vi "Load-Lookup Icon.vi"(8 "error in (no error)":errorcluster, 10 "Shell Icon":T1, 11 "TreeDirectory in":refnum<class "TreeDirectory.lvclass">) -> (0 "error out":errorcluster, 2 "Icon Index":i32, 3 "TreeDirectory (dup)":refnum<class "TreeDirectory.lvclass">)   [LabVIEW 2015, in "TreeDirectory.lvclass"]
uses:
  TreeDirectory.lvclass
  <vilib>/picture/picture.llb/imagedata.ctl
  TreeDirectory.lvclass/TreeDirectory.ctl
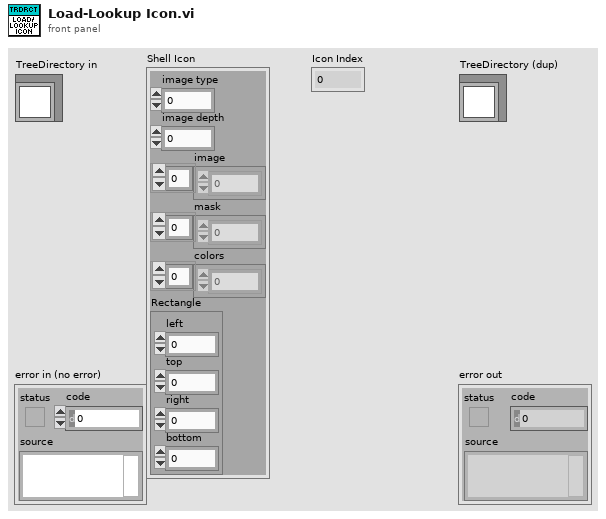
[diagram p1: front panel]
types:
  T1 = typedef "imagedata.ctl" = cluster{"image type":i32, "image depth":i32, "image":u8[], "mask":u8[], "colors":u32[], "Rectangle":cluster{"left":i16, "top":i16, "right":i16, "bottom":i16}}
  T2 = typedef "TreeDirectory.lvclass/State Data.ctl" = cluster{"IconLibrary":variant}
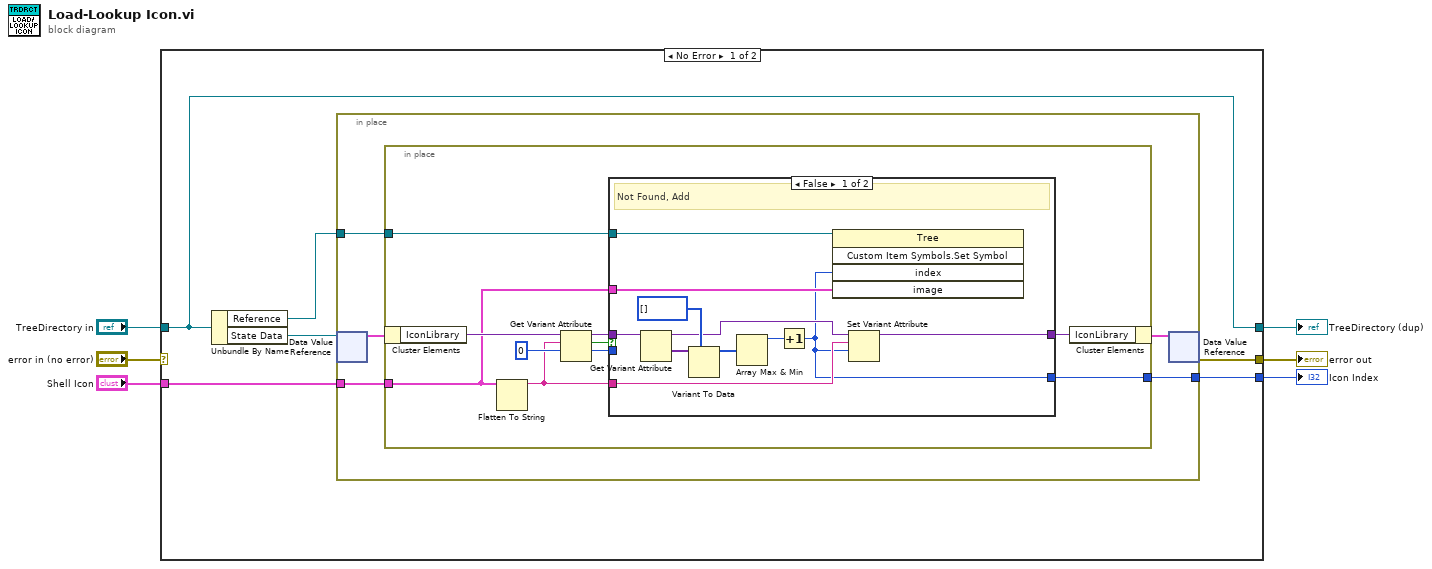
[diagram p0: block diagram]
diagram:
  n1 = case shown="No Error" "error in (no error)" {
    selector: "error in (no error)" -> [_ w42]
    tunnel: [w10 w42] -> w5
    tunnel: [w7 w41] -> w3
    tunnel: "TreeDirectory in" -> [w7 w41]
    tunnel: "Shell Icon" -> [w12 _]
    tunnel: [w11 _] -> w1
    frame No Error {
      n2 = Unbundle By Name(w7) -> ("Reference"=w8:refnum<vi>, "State Data"=w9:refnum<data-value>)
      n3 = in-place {
        in-place-border: w12 -> [w16]
        in-place-border: [w15] -> w11
        in-place-border: w8 -> [w13]
        n4 = in-place-dvr #1(w9) -> (w17:T2)  [unwired: 1 out]
        n5 = in-place {
          in-place-border: w16 -> [w19]
          in-place-border: [w21] -> w15
          in-place-border: w13 -> [w20]
          n6 = in-place-cluster #2(w17) -> ("IconLibrary"=w27:variant)
          n7 = Flatten To String(anything=w19) -> (data string=w18:string)  [unwired: 3 in, 2 out]
          n8 = Get Variant Attribute(Variant=w27, name=w18, default value (empty Variant)=0) -> (duplicate Variant=w24:variant, found=w25:bool, value=w22:i32)  [unwired: 1 in, 1 out]
          n9 = case shown="False" w25 {
            tunnel: w24 -> [w38 w40]
            tunnel: [w30 w40] -> w23
            tunnel: w22 -> [_ w39]
            tunnel: [w28 w39] -> w21
            tunnel: w20 -> [w33 _]
            tunnel: w19 -> [w32 _]
            tunnel: w18 -> [w29 _]
            frame False {
              # "Not Found, Add"
              n10 = Get Variant Attribute(Variant=w38) -> (duplicate Variant=w34:variant, values=w37:variant[])  [unwired: 3 in, 2 out]
              n11 = Variant To Data(type=i32[] [], Variant=w37) -> (data=w35:i32[])  [unwired: 1 in, 1 out]
              n12 = Array Max & Min(array=w35) -> (max value=w31:i32)  [unwired: 3 out]
              n13 = Increment(x=w31) -> (x+1=w28:i32)
              n14 = invoke class="Tree" method="Custom Item Symbols.Set Symbol"(reference=w33, "index"=w28, "image"=w32) -> ()  [unwired: 2 in, 5 out]
              n15 = Set Variant Attribute(Variant=w34, name=w29, value=w28) -> (Variant out=w30:variant)  [unwired: 1 in, 2 out]
            }
            frame True {
              # "Found, Pass Index"
            }
          }
          n16 = in-place-cluster #2("IconLibrary"=w23) -> (w14:T2)
        }
        n17 = in-place-dvr #1(w14) -> (w10:errorcluster)  [unwired: 1 out]
      }
    }
    frame Error {
    }
  }
  "error out" <- w5
  "TreeDirectory (dup)" <- w3
  "Icon Index" <- w1
